vi "compute_engine_CH0CH1.vi"(0 "CH1 POSITION":dbl step=0.001, 1 "CH2 POSITION":dbl step=0.001, 3 "Array In":u8[](array[numeric]), 4 "Input Select":u16(ring), 5 "INPUT1 range IN":u8, 8 "INPUT1 multiplier":dbl, 9 "Number of datapoints":dbl, 12 "INPUT2 multiplier":dbl, 13 "DC Filter":bool, 14 "INPUT1 shift":dbl, 15 "AC/DC INPUT2":bool, 16 "INPUT2 shift":dbl, 19 "AC /DC INPUT1":bool) -> (10 "Voltage":dbl[](array[numeric]), 17 "VRMS INPUT1":dbl format="%#.6g", 18 "Current":dbl[](array[numeric]), 20 "VDC INPUT2":dbl format="%#.6g", 21 "VRMS INPUT2":dbl format="%#.6g", 23 "Freq CH1 Hz":dbl format="%#.6g", 24 "VDC INPUT1":dbl format="%#.6g", 25 "Freq CH0 Hz":dbl format="%#.6g", 26 "Sig Out":dynamicdata(graph), 27 "RAW":dynamicdata(graph))   [LabVIEW 2012]
panel:
  out "CH1_OUT":dbl[](array[numeric])
  out "CH0_OUT":dbl[](array[numeric])
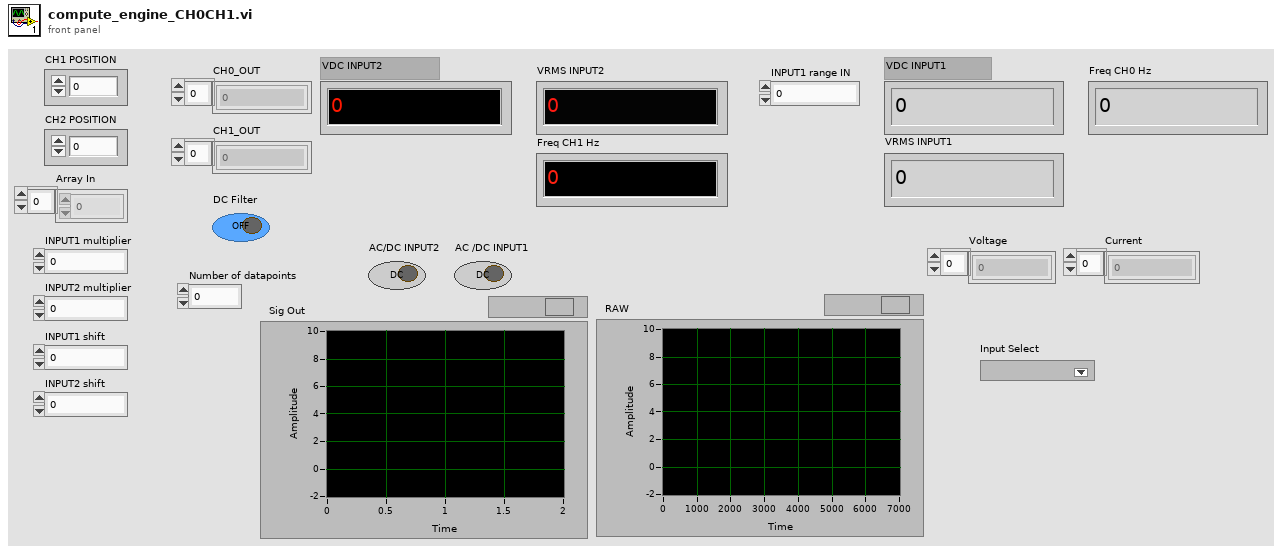
[diagram p1: front panel]
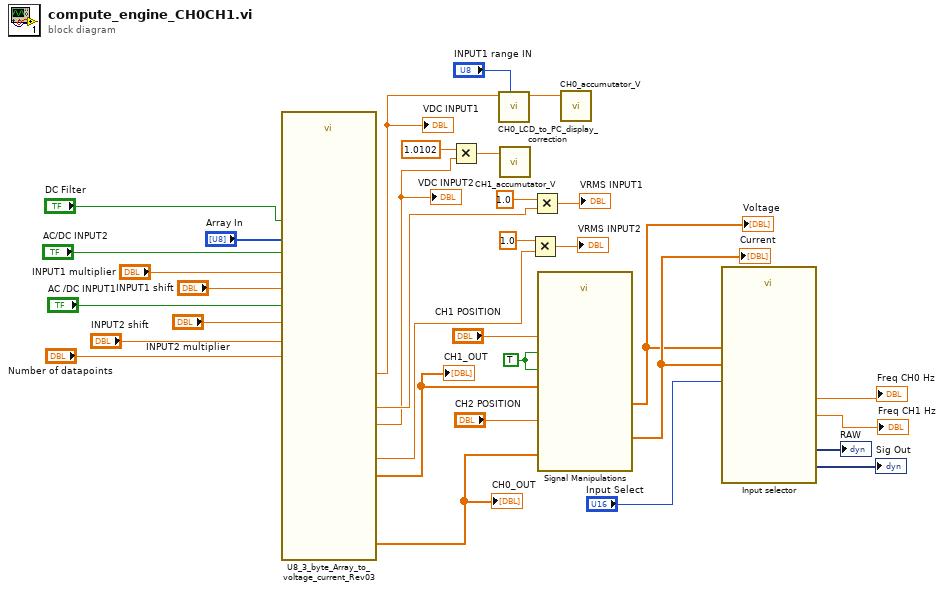
[diagram p0: block diagram]
diagram:
  w31 = TRUE
  n1 = call "U8_3_byte_Array_to_voltage_current_Rev03.vi"("Nmbr_of_datapoints"="Number of datapoints", "Array In"="Array In", "INPUT1 AC couple"="AC/DC INPUT2", "INPUT2 AC couple"="AC /DC INPUT1", "INPUT2 multiplier"="INPUT2 multiplier", "INPUT1 multiplier"="INPUT1 multiplier", "INPUT2 Shift V"="INPUT2 shift", "AC/DC"="DC Filter", "INPUT1 Shift V"="INPUT1 shift") -> ("INPUT1RMS"=w6:dbl, "INPUT2RMS"=w28:dbl, "INPUT1 Vave"=w2:dbl, "INPUT2 Vave"=w3:dbl, "Voltage"=w25:dbl[], "Current"=w24:dbl[])  [unwired: 5 out]
  "CH0_OUT" <- w25
  "CH1_OUT" <- w24
  "VDC INPUT2" <- w3
  "VDC INPUT1" <- w2
  n2 = Multiply(x=1.0102, y=w3) -> (x*y=w33:dbl)
  n3 = call "CH0_LCD_to_PC_display_correction.vi"("CH0_range_in"="INPUT1 range IN", "Vin"=w2) -> ("Vout"=w9:dbl)  [unwired: 9 in]
  n4 = call "CH1_accumutator_V.vi"("Vin"=w33) -> ()  [unwired: 10 in, 1 out]
  n5 = Multiply(x=1.0, y=w28) -> (x*y=→"VRMS INPUT2":dbl)
  n6 = Multiply(x=1.0, y=w6) -> (x*y=→"VRMS INPUT1":dbl)
  n7 = call "Signal Manipulations.vi"("CH1 Differential Mode"=w31, "CH0 Differential Mode"=w31, "CH1 POSITION"="CH2 POSITION", "CH1 IN"=w24, "CH0 POSITION"="CH1 POSITION", "CH0 IN"=w25) -> ("Current"=w5:dbl[], "Voltage"=w4:dbl[])  [unwired: 4 in]
  "Voltage" <- w4
  "Current" <- w5
  n8 = call "CH0_accumutator_V.vi"("Vin"=w9) -> ()  [unwired: 10 in, 1 out]
  n9 = call "Input selector.vi"("Voltage INPUT2"=w5, "Voltage INPUT1"=w4, "Ring"="Input Select") -> ("CH1 (Hz)"=→"Freq CH1 Hz":dbl, "CH0 (Hz)"=→"Freq CH0 Hz":dbl, "Sig Out"=→"Sig Out":dynamicdata, "RAW"=→"RAW":dynamicdata)  [unwired: 3 in, 2 out]
